vi "Write MAP DVR.vi"(8 "error in (no error)":errorcluster, 10 "MAP DVR":refnum<data-value>, 11 "Instr Exe Write to File in":refnum<class "Instr Exe Write to File.lvclass">) -> (0 "error out":errorcluster, 3 "Instr Exe Write to File out":refnum<class "Instr Exe Write to File.lvclass">)   [LabVIEW 2014, in "Controller.lvlib" / "Instr Exe Write to File.lvclass"]
uses:
  Instr Exe Write to File.lvclass
  Instr Exe Write to File.lvclass/Instr Exe Write to File.ctl
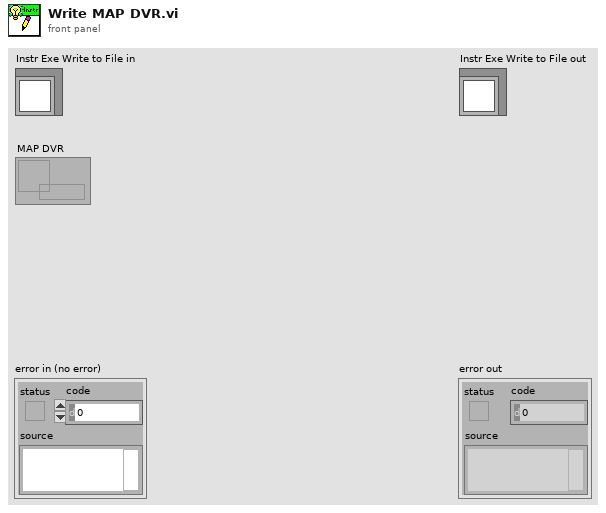
[diagram p1: front panel]
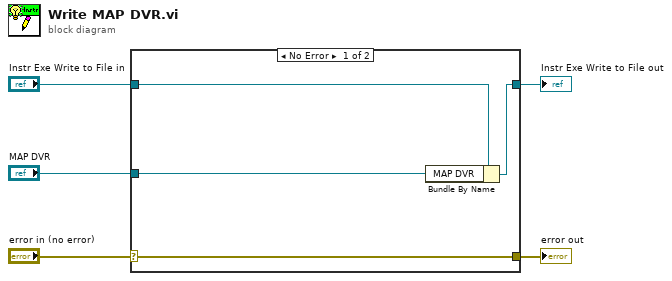
[diagram p0: block diagram]
diagram:
  n1 = case shown="No Error" "error in (no error)" {
    selector: "error in (no error)" -> [w9 w10]
    tunnel: [w9 w10] -> w4
    tunnel: [w7 w11] -> w2
    tunnel: "Instr Exe Write to File in" -> [w8 w11]
    tunnel: "MAP DVR" -> [w6 _]
    frame No Error {
      n2 = Bundle By Name(cluster=w8, "MAP DVR"=w6) -> (w7:refnum<class "Instr Exe Write to File.lvclass">)
    }
    frame Error {
    }
  }
  "error out" <- w4
  "Instr Exe Write to File out" <- w2
